vi "Temperature Warnings.vi"() -> ()   [LabVIEW 2012]
doc: "This VI uses a Case structure to determine and handle if a user has entered an invalid value. An Error case structure is also used to handle incoming errors."
panel:
  out "Warning Text":string="No Warning"
  out "Warning?":bool
  in  "Min Temperature":dbl
  in  "Max Temperature":dbl
  in  "Current Temperature":dbl
  out "Error Out":errorcluster
  in  "Error In":errorcluster
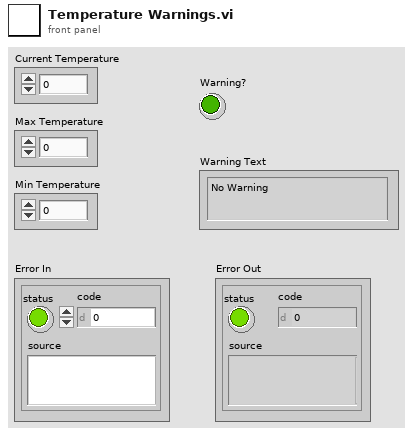
[diagram p1: front panel]
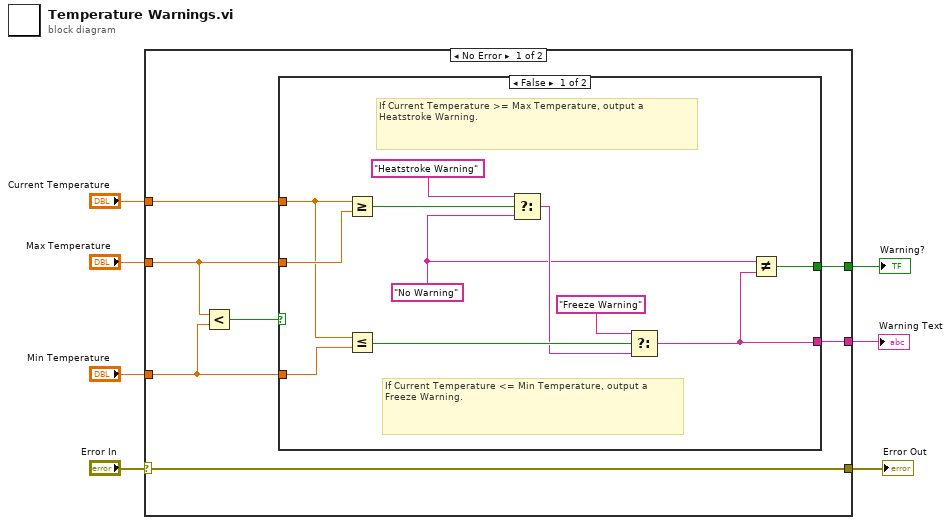
[diagram p0: block diagram]
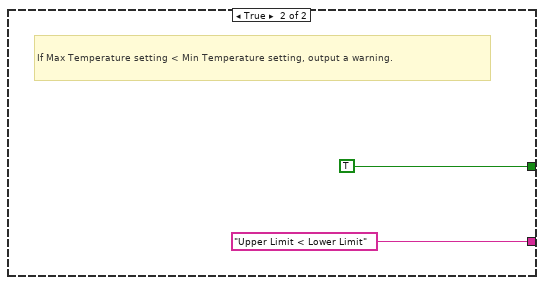
[diagram p2: hidden frame]
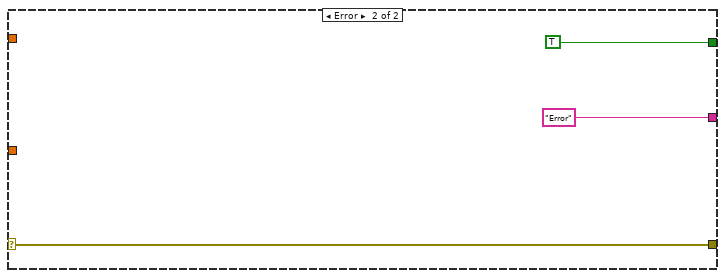
[diagram p3: hidden frame]
diagram:
  n1 = case shown="No Error" "Error In" {
    selector: "Error In" -> [w12 w30]
    tunnel: [w14 "Error" ("f")] -> w1
    tunnel: [w13 TRUE] -> w2
    tunnel: [w12 w30] -> w6
    tunnel: "Min Temperature" -> [w9 _]
    tunnel: "Current Temperature" -> [w11 _]
    tunnel: "Max Temperature" -> [w10 _]
    frame No Error {
      n2 = Less?(x=w10, y=w9) -> (x < y?=w8:bool)
      n3 = case shown="False" w8 {
        tunnel: [w15 "Upper Limit < Lower Limit" ("f")] -> w14
        tunnel: [w25 TRUE] -> w13
        tunnel: w10 -> [w24 _]
        tunnel: w9 -> [w21 _]
        tunnel: w11 -> [w17 _]
        frame False {
          w16 = "No Warning" ("f")
          # "If Current Temperature <= Min Temperature, output a Freeze Warning."
          # "If Current Temperature >= Max Temperature, output a Heatstroke Warning."
          n4 = Greater Or Equal?(x=w17, y=w24) -> (x >= y?=w23:bool)
          n5 = Less Or Equal?(x=w17, y=w21) -> (x <= y?=w19:bool)
          n6 = Select(t="Heatstroke Warning", s=w23, f=w16) -> (s? t:f=w18:string)
          n7 = Select(t="Freeze Warning", s=w19, f=w18) -> (s? t:f=w15:string)
          n8 = Not Equal?(x=w16, y=w15) -> (x != y?=w25:bool)
        }
        frame True {
          # "If Max Temperature setting < Min Temperature setting, output a warning."
        }
      }
    }
    frame Error {
    }
  }
  "Error Out" <- w6
  "Warning?" <- w2
  "Warning Text" <- w1
